vi "DSF.Engine.Pool.Plugin Interface.Set Plugin Interfaces.vi"(10 "Plugin Interfaces":refnum<class "DSF.Engine.Interface.Plugin.lvclass">[](array[class]), 11 "Plugin Interface Pool in":refnum<class "DSF.Engine.Pool.Plugin Interface.lvclass">) -> (3 "Plugin Interface Pool out":refnum<class "DSF.Engine.Pool.Plugin Interface.lvclass">)   [LabVIEW 2017, in "DSF.Engine.lvlib" / "DSF.Engine.Pool.Plugin Interface.lvclass"]
uses:
  DSF.Engine.Pool.Plugin Interface.lvclass
  Interface/DSF.Engine.Interface.Plugin.lvclass
  DSF.Engine.Pool.Plugin Interface.lvclass/DSF.Engine.Pool.Plugin Interface.ctl
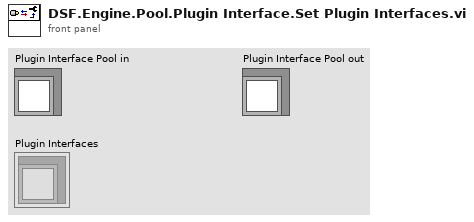
[diagram p1: front panel]
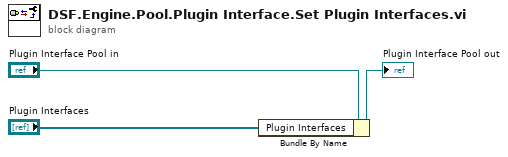
[diagram p0: block diagram]
diagram:
  n1 = Bundle By Name(cluster="Plugin Interface Pool in", "Plugin Interfaces"="Plugin Interfaces") -> (→"Plugin Interface Pool out":refnum<class "DSF.Engine.Pool.Plugin Interface.lvclass">)
